vi "FDM Cluster to NIVS Double Array.vi"(1 "Buffer In":dbl[](array[numeric]), 2 "Cluster":T1={"Version"={"version"=20, "pad"=0}, "Positions"={"Doubles"={"longitude"=0.0, "latitude"=0.0, "altitude"=0.0}, "Singles"={"agl"=0.0, "phi"=0.0, "theta"=0.0, "psi"=0.0, "alpha"=0.0, "beta"=0.0}}, "Velocities"={"phidot"=0.0, "thetadot"=0.0, "psidot"=0.0, "vcas"=0.0, "climb_rate"=0.0, "v_north"=0.0, "v_east"=0.0, "v_down"=0.0, "v_wind_body_north"=0.0, "v_wind_body_east"=0.0, "v_wind_body_down"=0.0}, "Accelerations"={"A_X_pilot"=0.0, "A_Y_pilot"=0.0, "A_Z_pilot"=0.0}, "Stall"={"stall_warning"=0.0, "slip_deg"=0.0}, "Engine Status"={"num_engines"=0, "eng_state"=[0, 0, 0, 0], "rpm"=[0.0, 0.0, 0.0, 0.0], "fuel_flow"=[0.0, 0.0, 0.0, 0.0], "fuel_px"=[0.0, 0.0, 0.0, 0.0], "egt"=[0.0, 0.0, 0.0, 0.0], "cht"=[0.0, 0.0, 0.0, 0.0], "mp_osi"=[0.0, 0.0, 0.0, 0.0], "tit"=[0.0, 0.0, 0.0, 0.0], "oil_temp"=[0.0, 0.0, 0.0, 0.0], "oil_px"=[0.0, 0.0, 0.0, 0.0]}, "Consumables"={"num_tanks"=0, "fuel_quantity"=[0.0, 0.0, 0.0, 0.0]}, "Gear Status"={"num_wheels"=0, "wow"=[0, 0, 0, 0], "gear_pos"=[0.0, 0.0, 0.0, 0.0], "gear_steer"=[0.0, 0.0, 0.0, 0.0], "gear_compression"=[0.0, 0.0, 0.0, 0.0]}, "Environment"={"curr_time"=0, "warp"=0, "visibility"=0.0}, "Control Surface Positions"={"elevator"=0.0, "elevator_trim_tab"=0.0, "left_flap"=0.0, "right_flap"=0.0, "left aileron"=0.0, "right_aileron"=0.0, "rudder"=0.0, "nose_wheel"=0.0, "speedbrake"=0.0, "spoilers"=0.0}}) -> (0 "DBL Array":dbl[](array[numeric]))   [LabVIEW 2010, in "Flight Gear Data Custom Device.lvlib"]
uses:
  Flight Gear Data Custom Device.lvlib
  FGNetFDM.ctl
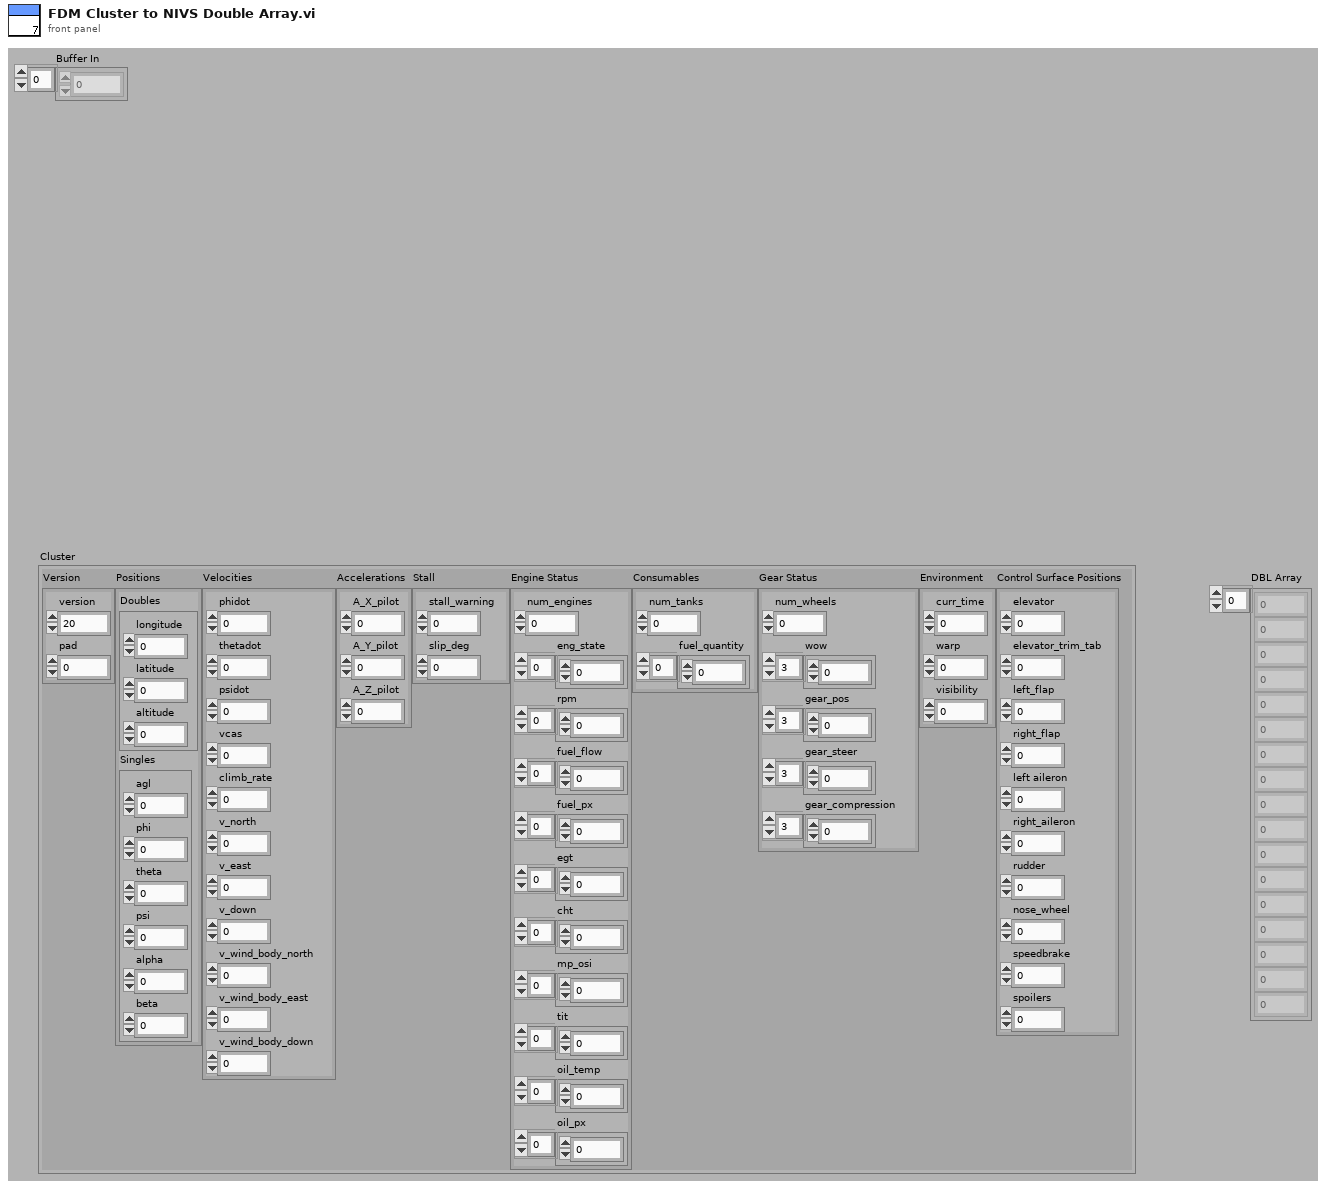
[diagram p1: front panel]
types:
  T1 = typedef "Flight Gear Data Custom Device.lvlib/FGNetFDM.ctl" = cluster{"Version":cluster{"version":u32, "pad":u32}, "Positions":cluster{"Doubles":cluster{"longitude":dbl, "latitude":dbl, "altitude":dbl}, "Singles":cluster{"agl":sgl, "phi":sgl, "theta":sgl, "psi":sgl, "alpha":sgl, "beta":sgl}}, "Velocities":cluster{"phidot":sgl, "thetadot":sgl, "psidot":sgl, "vcas":sgl, "climb_rate":sgl, "v_north":sgl, "v_east":sgl, "v_down":sgl, "v_wind_body_north":sgl, "v_wind_body_east":sgl, "v_wind_body_down":sgl}, "Accelerations":cluster{"A_X_pilot":sgl, "A_Y_pilot":sgl, "A_Z_pilot":sgl}, "Stall":cluster{"stall_warning":sgl, "slip_deg":sgl}, "Engine Status":cluster{"num_engines":u32, "eng_state":u32[], "rpm":sgl[], "fuel_flow":sgl[], "fuel_px":sgl[], "egt":sgl[], "cht":sgl[], "mp_osi":sgl[], "tit":sgl[], "oil_temp":sgl[], "oil_px":sgl[]}, "Consumables":cluster{"num_tanks":u32, "fuel_quantity":sgl[]}, "Gear Status":cluster{"num_wheels":u32, "wow":u32[], "gear_pos":sgl[], "gear_steer":sgl[], "gear_compression":sgl[]}, "Environment":cluster{"curr_time":u32, "warp":i32, "visibility":sgl}, "Control Surface Positions":cluster{"elevator":sgl, "elevator_trim_tab":sgl, "left_flap":sgl, "right_flap":sgl, "left aileron":sgl, "right_aileron":sgl, "rudder":sgl, "nose_wheel":sgl, "speedbrake":sgl, "spoilers":sgl}}
  T2 = cluster{"longitude":dbl, "latitude":dbl, "altitude":dbl}
  T3 = cluster{"agl":sgl, "phi":sgl, "theta":sgl, "psi":sgl, "alpha":sgl, "beta":sgl}
  T4 = cluster{"phidot":sgl, "thetadot":sgl, "psidot":sgl, "vcas":sgl, "climb_rate":sgl, "v_north":sgl, "v_east":sgl, "v_down":sgl, "v_wind_body_north":sgl, "v_wind_body_east":sgl, "v_wind_body_down":sgl}
  T5 = cluster{"A_X_pilot":sgl, "A_Y_pilot":sgl, "A_Z_pilot":sgl}
  T6 = cluster{"elevator":sgl, "elevator_trim_tab":sgl, "left_flap":sgl, "right_flap":sgl, "left aileron":sgl, "right_aileron":sgl, "rudder":sgl, "nose_wheel":sgl, "speedbrake":sgl, "spoilers":sgl}
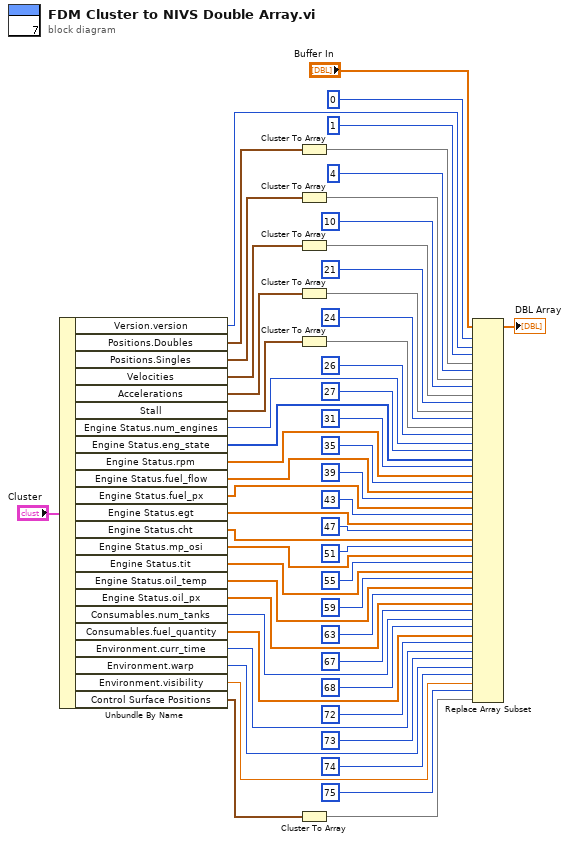
[diagram p0: block diagram]
diagram:
  n1 = Unbundle By Name("Cluster") -> ("Version.version"=w54:u32, "Positions.Doubles"=w52:T2, "Positions.Singles"=w51:T3, "Velocities"=w50:T4, "Accelerations"=w49:T5, "Stall"=w46:cluster{"stall_warning":sgl, "slip_deg":sgl}, "Engine Status.num_engines"=w45:u32, "Engine Status.eng_state"=w44:u32[], "Engine Status.rpm"=w43:sgl[], "Engine Status.fuel_flow"=w42:sgl[], "Engine Status.fuel_px"=w41:sgl[], "Engine Status.egt"=w40:sgl[], "Engine Status.cht"=w39:sgl[], "Engine Status.mp_osi"=w38:sgl[], "Engine Status.tit"=w37:sgl[], "Engine Status.oil_temp"=w36:sgl[], "Engine Status.oil_px"=w35:sgl[], "Consumables.num_tanks"=w34:u32, "Consumables.fuel_quantity"=w33:sgl[], "Environment.curr_time"=w32:u32, "Environment.warp"=w31:i32, "Environment.visibility"=w30:sgl, "Control Surface Positions"=w2:T6)
  n2 = Cluster To Array(cluster=w52) -> (array=w11:dbl[])
  n3 = Cluster To Array(cluster=w51) -> (array=w9:sgl[])
  n4 = Cluster To Array(cluster=w50) -> (array=w8:sgl[])
  n5 = Cluster To Array(cluster=w49) -> (array=w48:sgl[])
  n6 = Cluster To Array(cluster=w46) -> (array=w47:sgl[])
  n7 = Cluster To Array(cluster=w2) -> (array=w1:sgl[])
  n8 = Replace Array Subset(array="Buffer In", new element #1=w54, index #1=0 ("index"), new element #2=w11, index #2=1 ("index"), new element #3=w9, index #3=4 ("index"), new element #4=w8, index #4=10 ("index"), new element #5=w48, index #5=21 ("index"), new element #6=w47, index #6=24 ("index"), new element #7=w45, index #7=26 ("index"), new element #8=w44, index #8=27 ("index 2"), new element #9=w43, index #9=31 ("index 3"), new element #10=w42, index #10=35 ("index 4"), new element #11=w41, index #11=39 ("index 5"), new element #12=w40, index #12=43 ("index 6"), new element #13=w39, index #13=47 ("index 7"), new element #14=w38, index #14=51 ("index 8"), new element #15=w37, index #15=55 ("index 9"), new element #16=w36, index #16=59 ("index 10"), new element #17=w35, index #17=63 ("index 11"), new element #18=w34, index #18=67 ("index 12"), new element #19=w33, index #19=68 ("index 13"), new element #20=w32, index #20=72 ("index 14"), new element #21=w31, index #21=73 ("index 15"), new element #22=w30, index #22=74 ("index 16"), new element #23=w1, index #23=75 ("index 16")) -> (→"DBL Array":dbl[])
